vi "RSZVB Set Automatic Generator Attenuator.vi"(7 "Automatic Attenuation (F: Off)":bool=TRUE, 8 "error in (no error)":errorcluster {"code" format="%.0x"}, 9 "Port (1)":i32=1, 10 "Channel (1)":i32=1, 11 "VISA session":refnum<visa-resource-name>) -> (0 "error out":errorcluster {"code" format="%.0x"}, 3 "dup VISA session":refnum<visa-resource-name>)   [LabVIEW 2011]
doc: "This VI sets whether the attenuation factor for the generated wave at test port no. <Pt> is set manually or automatically. \n\nNote(s):\n\n(1) This VI can be used only with R&S ZVA and ZVB instruments.\n\nRemote-control command(s):\nSOURce<Ch>:POWer<Pt>:ATTenuation:AUTO ON | OFF"
uses:
  _utility/RSZVB Global Data.vi
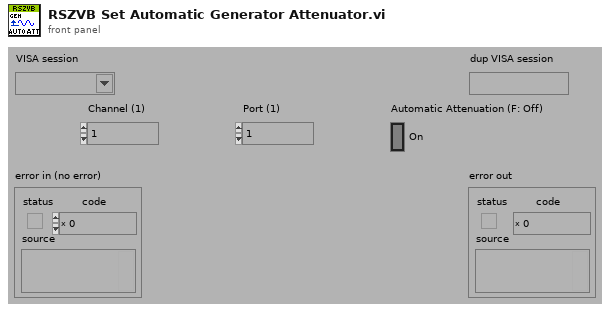
[diagram p1: front panel]
types:
  T1 = cluster{"Error Checking (T: On)":bool, "Installed Options":string[], "Data Valid?":bool, "Ports":i32, "Model":string[], "Option Checking (T: On)":bool}[]
  T2 = cluster{"Error Checking (T: On)":bool, "Installed Options":string[], "Data Valid?":bool, "Ports":i32, "Model":string[], "Option Checking (T: On)":bool}
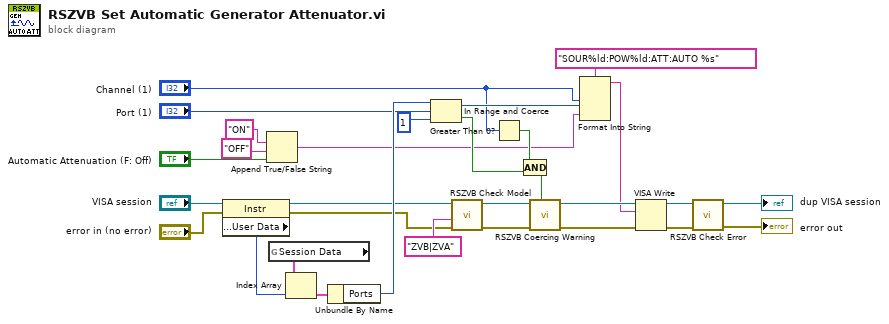
[diagram p0: block diagram]
diagram:
  n1 = property class="Instr"(reference="VISA session", error in="error in (no error)") -> (reference out=w15:refnum<visa-resource-name>, error out=w14:errorcluster, "General Settings:User Data"=w17:u32)
  n2 = Append True/False String(1:"Automatic Attenuation (F: Off)", 2:"OFF", 3:"ON") -> (0:w1:string)  [unwired: 1 in]
  n3 = global read "RSZVB Global Data.vi" "Session Data"() -> (w18:T1)
  n4 = Index Array(array=w18, index=w17) -> (element=w19:T2)
  n5 = Unbundle By Name(w19) -> ("Ports"=w16:i32)
  n6 = In Range and Coerce(upper limit=w16, x="Port (1)", lower limit=1) -> (coerced(x)=w12:i32, In Range?=w13:bool)
  n7 = call "RSZVB Check Model.vi"("error in (no error)"=w14, "Model"="ZVB|ZVA" ("Options"), "VISA session"=w15) -> ("error out"=w22:errorcluster, "dup VISA session"=w21:refnum<visa-resource-name>)  [unwired: 7 in]
  n8 = Greater Than 0?(x="Channel (1)") -> (x > 0?=w23:bool)
  n9 = Compound Arithmetic op=AND(w23, w13) -> (w25:bool)
  n10 = call "RSZVB Coercing Warning.vi"("In Range?"=w25, "error in (no error)"=w22, "VISA session"=w21) -> ("error out"=w28:errorcluster, "dup VISA session"=w29:refnum<visa-resource-name>)  [unwired: 7 in]
  n11 = Format Into String(format string="SOUR%ld:POW%ld:ATT:AUTO %s", "Channel (1)", w12, w1) -> (resulting string=w24:string)  [unwired: 2 in, 1 out]
  n12 = VISA Write(VISA resource name=w29, write buffer=w24, error in (no error)=w28) -> (VISA resource name out=w26:refnum<visa-resource-name>, error out=w27:errorcluster)  [unwired: 1 out]
  n13 = call "RSZVB Check Error.vi"("error in (no error)"=w27, "VISA session"=w26) -> ("error out"=→"error out":errorcluster, "dup VISA session"=→"dup VISA session":refnum<visa-resource-name>)  [unwired: 8 in]
